vi "FindeArrayIndexNullstelle.vi"(10 "Array":dbl[](array[numeric])) -> (2 "Array Index Nullstelle":i32)   [LabVIEW 2016]
doc: "Bestimmt den Index eines Nulldurchgangs innerhalb eines Arrays mit Messwerten eines periodischen Signals. Dabei wird die erste Nullstelle ausgegeben die gefunden wurde!"
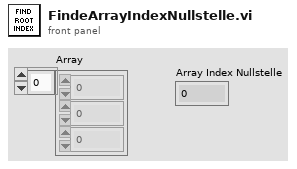
[diagram p1: front panel]
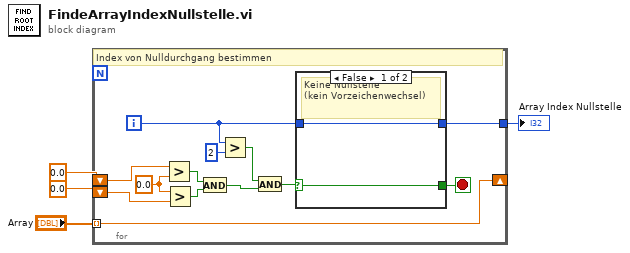
[diagram p0: block diagram]
diagram:
  n1 = for {
    tunnel: "Array" -> [w17] mode=indexing
    shift-right: [w17] -> _
    shift-left: 0.0 ("Numeric") -> [w16]
    shift-left: 0.0 ("Numeric") -> [w14]
    tunnel: [w10] -> w1
    i -> [w6]
    stop <- w11 stop-if-true
    w15 = 0.0 ("y")
    # "Index von Nulldurchgang bestimmen"
    n2 = Greater?(x=w16, y=w15) -> (0:w12:bool)
    n3 = Greater?(x=w15, y=w14) -> (0:w13:bool)
    n4 = And(x=w12, y=w13) -> (x .and. y?=w8:bool)
    n5 = Greater?(x=w6, y=2) -> (0:w7:bool)
    n6 = And(x=w7, y=w8) -> (x .and. y?=w9:bool)
    n7 = case shown="False" w9 {
      selector: w9 -> [w19 w21]
      tunnel: w6 -> [w18 w20]
      tunnel: [w19 w21] -> w11
      tunnel: [w18 w20] -> w10
      frame False {
        # "Keine Nullstelle\n(kein Vorzeichenwechsel)"
      }
      frame True {
        # "Nullstelle\n(Vorzeichenwechsel)"
      }
    }
  }
  "Array Index Nullstelle" <- w1
